vi "HAL camera initialize.vi"(7 "Select camera model(s)":string[](array[string])) -> (1 "error out":errorcluster)   [LabVIEW 2015]
panel:
  in  "Quit":bool
  in  "Select Camera Number":u16(ring) items=["*** Please wait ***"=1]
  out "Cameras Avalable":T1(array[cluster])
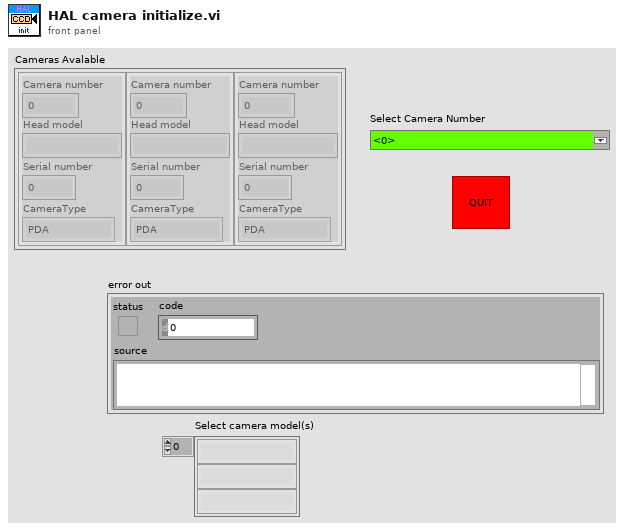
[diagram p1: front panel]
types:
  T1 = cluster{"Camera number":i32, "Head model":string, "Serial number":i32, "CameraType":enum32{"PDA", "iXon", "ICCD", "EMCCD", "CCD", "iStar", "third party camera", "iDus", "Newton", "Surcam", "USB ICCD", "Luca", "Reserved", "iKon", "InGaAs", "iVac", "Unprogrammed", "Clara", "USB iStar", "SimCam", "Neo", "iXon Ultra", "Volmos", "iVac Ultra"}}[]
  T2 = enum8{"Enabled", "Disabled", "Disabled and Grayed Out"}
  T3 = cluster{"Camera number":i32, "Head model":string, "Serial number":i32, "CameraType":enum32{"PDA", "iXon", "ICCD", "EMCCD", "CCD", "iStar", "third party camera", "iDus", "Newton", "Surcam", "USB ICCD", "Luca", "Reserved", "iKon", "InGaAs", "iVac", "Unprogrammed", "Clara", "USB iStar", "SimCam", "Neo", "iXon Ultra", "Volmos", "iVac Ultra"}}
  T4 = typedef "AndorCapabilities typedef.ctl" = cluster{"AcqModes":cluster{"single":bool, "video":bool, "accumulate":bool, "kinetic":bool, "frametransfer":bool, "fastkinetics":bool}, "ReadModes":cluster{"fullimage":bool, "subimage":bool, "singletrack":bool, "fvb":bool, "multitrack":bool, "randomtrack":bool}, "TriggerModes":cluster{"internal":bool, "external":bool}, "CameraType":enum32{"PDA", "iXon", "ICCD", "EMCCD", "CCD", "iStar", "third party camera"}, "PixelMode":cluster{"8-bit":bool, "14-bit":bool, "16-bit":bool, "32-bit":bool, "color mode":enum16{"Mono", "RGB", "CMY"}}, "SetFunctions":cluster{"vreadout":bool, "hreadout":bool, "temperature":bool, "gain":bool, "emccdgain":bool}, "GetFunctions":cluster{"temperature":bool, "targettemperature":bool, "temperaturerange":bool, "detectorsize":bool, "gain":bool, "emccdgain":bool}, "Features":cluster{"polling":bool, "events":bool, "spooling":bool, "shutter":bool}}
  T5 = enum32{"PDA", "iXon", "ICCD", "EMCCD", "CCD", "iStar", "third party camera"}
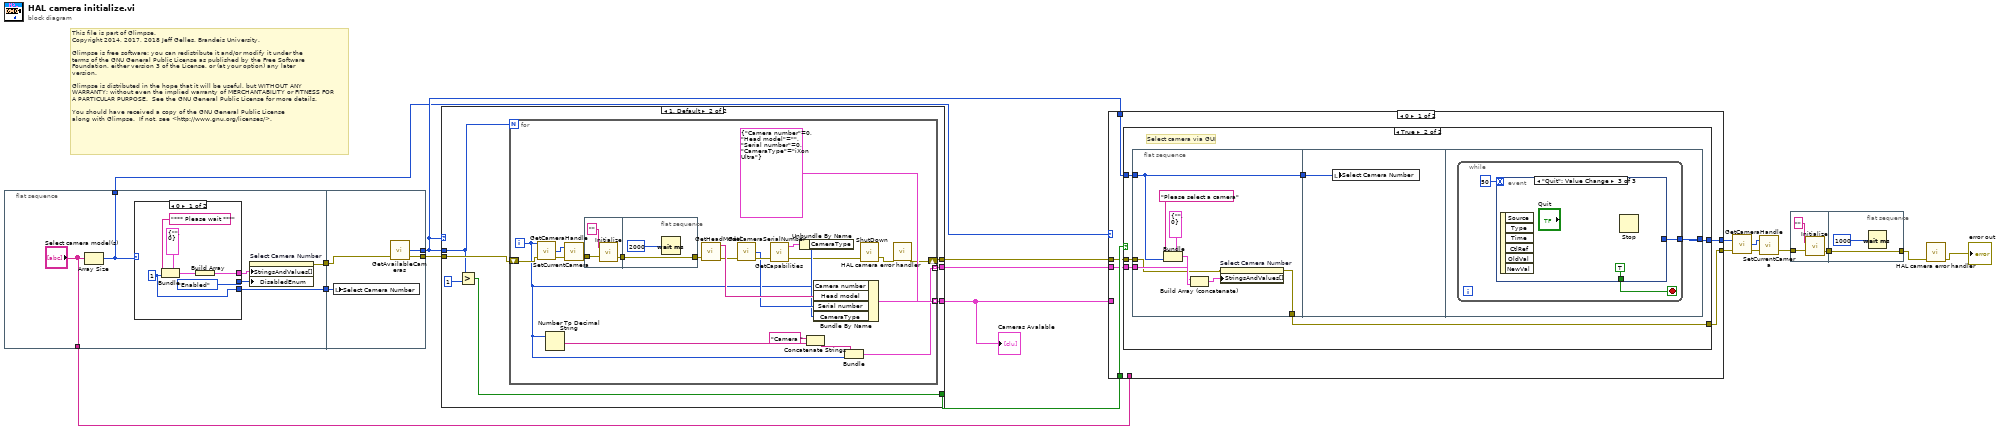
[diagram p0: block diagram]
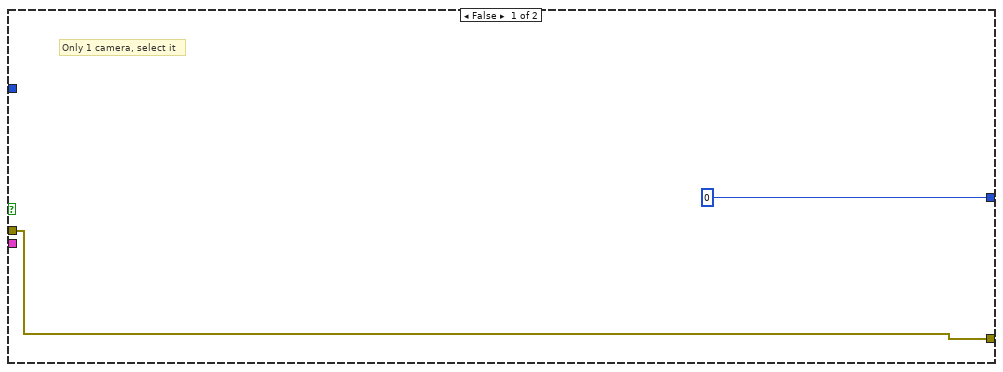
[diagram p2: hidden frame]
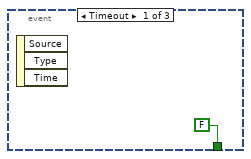
[diagram p3: hidden frame]
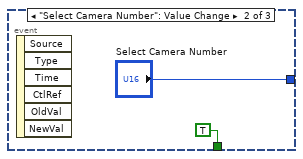
[diagram p4: hidden frame]
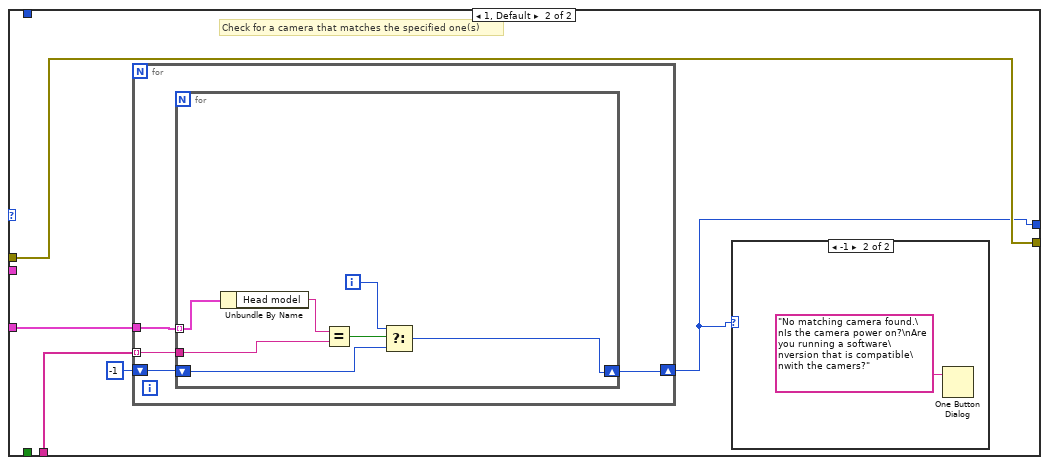
[diagram p5: hidden frame]
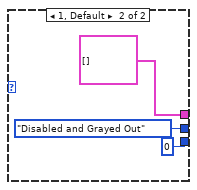
[diagram p7: hidden frame]
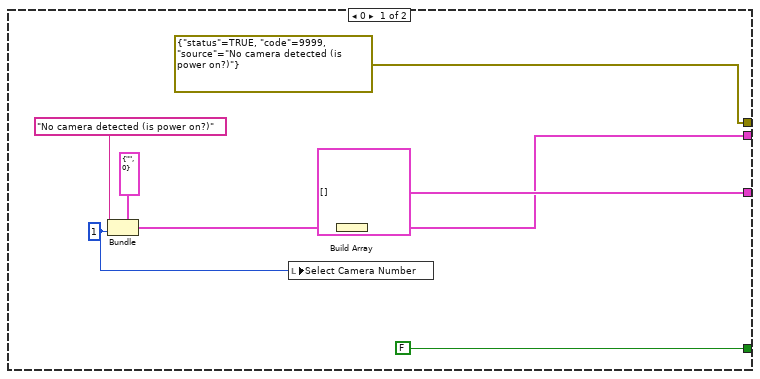
[diagram p8: hidden frame]
diagram:
  # "This file is part of Glimpse. \nCopyright 2014, 2017, 2018 Jeff Gelles, Brandeis University.    \n\nGlimpse is free software: you can redistribute it and/or modify it under the \nterms of the GNU General Public License as published by the Free Software \nFoundation, either version 3 of the License, or (at your option) any later \nversion.\n\nGlimpse is distributed in the hope that it will be useful, but WITHOUT ANY \nWARRANTY; without even the implied warranty of MERCHANTABILITY or FITNESS FOR \nA PARTICULAR PURPOSE.  See the GNU General Public License for more details.\n\nYou should have received a copy of the GNU General Public License\nalong with Glimpse.  If not, see <http://www.gnu.org/licenses/>."
  n1 = flat-sequence {
    tunnel: [w23] -> w12
    tunnel: [w22] -> w10
    tunnel: [w20] -> w7
    tunnel: ["Select camera model(s)"] -> w5
    tunnel: [w37] -> w18
    tunnel: [w36] -> w13
    tunnel: w12 -> [w34]
    tunnel: w10 -> [w35]
    frame #0 {
      n2 = Array Size(array="Select camera model(s)") -> (size(s)=w20:i32)
      n3 = case shown="0" w20 {
        tunnel: [w27 cluster{string, i32}[] []] -> w24
        tunnel: [w26 0] -> w22
        tunnel: [T2."Enabled" ("Disabled") T2."Disabled and Grayed Out" ("Disabled")] -> w21
        frame 0 {
          w26 = 1
          n4 = Bundle(cluster=cluster{string, i32} {"", 0}, "*** Please wait ***", w26) -> (w28:cluster{string, i32})
          n5 = Build Array(w28) -> (w27:cluster{string, i32}[])
        }
        frame 1, Default {
        }
      }
      n6 = property on="Select Camera Number" class="Ring (strict)"("StringsAndValues[]"=w24, "DisabledEnum"=w21) -> (error out=w23:errorcluster)  [unwired: 2 in, 1 out]
    }
    frame #1 {
      n7 = local write "Select Camera Number"(w35) -> ()
      n8 = call <userlib>:"GetAvailableCameras.vi"("error in (no error)"=w34) -> ("error out"=w37:errorcluster, "totalCameras"=w36:i32)  [unwired: 2 in, 1 out]
    }
  }
  n9 = case shown="1, Default" w13 {
    tunnel: w18 -> [_ w51]
    tunnel: [T1 [] w50] -> w6
    tunnel: [errorcluster {"status"=TRUE, "code"=9999, "source"="No camera detected (is power on?)"} ("error constant") w49] -> w8
    tunnel: [FALSE w48] -> w17
    tunnel: [w40 w47] -> w9
    tunnel: w13 -> [_ w46]
    frame 0 {
      w39 = 1
      n10 = Bundle(cluster=cluster{string, i32} {"", 0}, "No camera detected (is power on?)", w39) -> (w41:cluster{string, i32})
      n11 = local write "Select Camera Number"(w39) -> ()
      n12 = Build Array(w41) -> (w40:cluster{string, i32}[])
    }
    frame 1, Default {
      n13 = Greater?(x=w46, y=1) -> (0:w48:bool)
      n14 = for {
        N: w46 -> [_]
        shift-right: [w53] -> w49
        shift-left: w51 -> [w74]
        tunnel: [w66] -> w50 mode=indexing
        tunnel: [w62] -> w47 mode=indexing
        i -> [w63]
        n15 = call <userlib>:"GetCameraHandle.vi"("error in (no error)"=w74, "cameraIndex"=w63) -> ("error out"=w73:errorcluster, "cameraHandle"=w71:i32)  [unwired: 1 in, 1 out]
        n16 = Number To Decimal String(number=w63) -> (decimal integer string=w64:string)  [unwired: 1 in]
        n17 = call <userlib>:"SetCurrentCamera.vi"("error in (no error)"=w73, "cameraHandle"=w71) -> ("error out"=w58:errorcluster)  [unwired: 1 out]
        n18 = flat-sequence {
          tunnel: w58 -> [w77]
          tunnel: [w76] -> w56
          tunnel: [w79] -> w57
          tunnel: w56 -> [w79]
          frame #0 {
            n19 = call <userlib>:"Initialize.vi"("error in (no error)"=w77, "directory (\"\")"="" ("directory (\"\")")) -> ("error out"=w76:errorcluster)  [unwired: 1 out]
          }
          frame #1 {
            n20 = Wait (ms)(milliseconds to wait=u32 2000) -> ()  [unwired: 1 out]
          }
        }
        n21 = call <userlib>:"GetHeadModel.vi"("error in (no error)"=w57) -> ("error out"=w59:errorcluster, "model"=w69:string)  [unwired: 2 in, 1 out]
        n22 = call <userlib>:"GetCameraSerialNumber.vi"("error in (no error)"=w59) -> ("error out"=w72:errorcluster, "number"=w68:i32)  [unwired: 2 in, 1 out]
        n23 = call <userlib>:"GetCapabilities.vi"("error in (no error)"=w72) -> ("error out"=w54:errorcluster, "caps"=w70:T4)  [unwired: 2 in, 1 out]
        n24 = Unbundle By Name(w70) -> ("CameraType"=w67:T5)
        n25 = Concatenate Strings("Camera " ("string"), w64) -> (w61:string)
        n26 = Bundle By Name(cluster=T3 {"Camera number"=0, "Head model"="", "Serial number"=0, "CameraType"=enum."iXon Ultra"} ("input cluster"), "Camera number"=w63, "Head model"=w69, "Serial number"=w68, "CameraType"=w67) -> (w66:T3)
        n27 = Bundle(w61, w63) -> (w62:cluster{string, i32})  [unwired: 1 in]
        n28 = call <userlib>:"ShutDown.vi"("error in (no error)"=w54) -> ("error out"=w55:errorcluster)  [unwired: 1 in, 1 out]
        n29 = call "HAL camera error handler.vi"("error in (no error)"=w55) -> ("error out"=w53:errorcluster)  [unwired: 10 in]
      }
    }
  }
  "Cameras Avalable" <- w6
  n30 = case shown="0" w7 {
    tunnel: w17 -> [w85 _]
    tunnel: [w84 w111] -> w16
    tunnel: w13 -> [w83 _]
    tunnel: [w82 w113] -> w11
    tunnel: w9 -> [w81 _]
    tunnel: w8 -> [w80 w113]
    tunnel: w6 -> [_ w115]
    tunnel: w5 -> [_ w114]
    frame 0 {
      n31 = case shown="True" w85 {
        tunnel: w83 -> [_ w93]
        tunnel: [u16 0 ("Select Camera Number") w92] -> w84
        tunnel: [w86 w90] -> w82
        tunnel: w81 -> [_ w89]
        tunnel: w80 -> [w86 w88]
        frame False {
          # "Only 1 camera, select it"
        }
        frame True {
          # "Select camera via GUI"
          n32 = flat-sequence {
            tunnel: w93 -> [w98]
            tunnel: [w98] -> w91
            tunnel: [w95] -> w90
            tunnel: w89 -> [w97]
            tunnel: w88 -> [w96]
            tunnel: w91 -> [w102]
            tunnel: [w103] -> w92
            frame #0 {
              n33 = Bundle(cluster=cluster{string, i32} {"", 0}, "Please select a camera", w98) -> (w100:cluster{string, i32})
              n34 = Build Array (concatenate)(w97, w100) -> (w94:cluster{string, i32}[])
              n35 = property on="Select Camera Number" class="Ring (strict)"(error in=w96, "StringsAndValues[]"=w94) -> (error out=w95:errorcluster)  [unwired: 1 in, 1 out]
            }
            frame #1 {
              n36 = local write "Select Camera Number"(w102) -> ()
            }
            frame #2 {
              n37 = while {
                tunnel: [w104] -> w103
                stop <- w105 stop-if-true
                n38 = event shown="[2] \"Quit\": Value Change" {
                  selector: _ -> [_ _ _]
                  dyn-events: _ -> [_ _ _]
                  timeout: 50 -> [_ _ _]
                  tunnel: [FALSE TRUE TRUE] -> w105
                  tunnel: [_ "Select Camera Number" _] -> w104
                  event Timeout {
                    n39 = event-data() -> ()  [unwired: 1 in, 3 out]
                  }
                  event "Select Camera Number": Value Change {
                    n40 = event-data() -> ()  [unwired: 1 in, 6 out]
                  }
                  event "Quit": Value Change {
                    n41 = event-data() -> ()  [unwired: 1 in, 6 out]
                    n42 = Stop() -> ()  [unwired: 1 in]
                  }
                }
              }
            }
          }
        }
      }
    }
    frame 1, Default {
      # "Check for a camera that matches the specified one(s)"
      n43 = for {
        tunnel: w115 -> [w120]
        tunnel: w114 -> [w119] mode=indexing
        shift-right: [w118] -> w111
        shift-left: -1 -> [w117]
        n44 = for {
          tunnel: w120 -> [w126] mode=indexing
          tunnel: w119 -> [w127]
          shift-right: [w122] -> w118
          shift-left: w117 -> [w121]
          i -> [w123]
          n45 = Unbundle By Name(w126) -> ("Head model"=w125:string)
          n46 = Equal?(x=w125, y=w127) -> (x = y?=w124:bool)
          n47 = Select(t=w123, s=w124, f=w121) -> (s? t:f=w122:i32)
        }
      }
      n48 = case shown="-1" w111 {
        frame 0, Default {
        }
        frame -1 {
          n49 = One Button Dialog(message="No matching camera found.\nIs the camera power on?\nAre you running a software\nversion that is compatible\nwith the camers?") -> ()  [unwired: 1 in, 1 out]
        }
      }
    }
  }
  n50 = call <userlib>:"GetCameraHandle.vi"("error in (no error)"=w11, "cameraIndex"=w16) -> ("error out"=w14:errorcluster, "cameraHandle"=w15:i32)  [unwired: 1 in, 1 out]
  n51 = call <userlib>:"SetCurrentCamera.vi"("error in (no error)"=w14, "cameraHandle"=w15) -> ("error out"=w3:errorcluster)  [unwired: 1 out]
  n52 = flat-sequence {
    tunnel: w3 -> [w130]
    tunnel: [w129] -> w4
    tunnel: [w132] -> w2
    tunnel: w4 -> [w132]
    frame #0 {
      n53 = call <userlib>:"Initialize.vi"("error in (no error)"=w130, "directory (\"\")"="" ("directory (\"\")")) -> ("error out"=w129:errorcluster)  [unwired: 1 out]
    }
    frame #1 {
      n54 = Wait (ms)(milliseconds to wait=u32 1000) -> ()  [unwired: 1 out]
    }
  }
  n55 = call "HAL camera error handler.vi"("error in (no error)"=w2) -> ("error out"=→"error out":errorcluster)  [unwired: 10 in]
